vi "Hybrid Get Control Status.vi"(8 "error in (no error)":errorcluster, 11 "VI in":refnum<vi>) -> (0 "error out":errorcluster, 1 "Pause":bool, 2 "Ramp":bool, 3 "VI out":refnum<vi>, 5 "Slew Rate [A/s]":dbl format="%.1f", 7 "Setpoint":dbl format="%.2f")   [LabVIEW 2019]
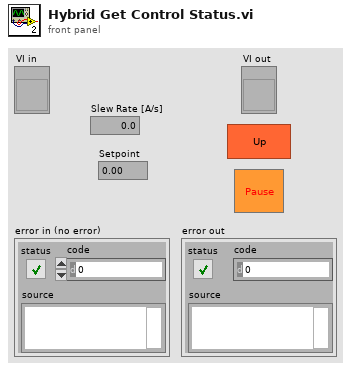
[diagram p1: front panel]
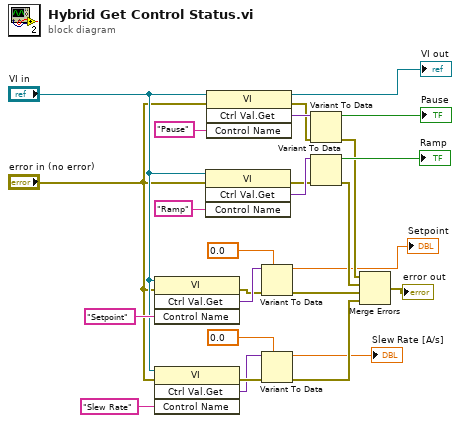
[diagram p0: block diagram]
diagram:
  n1 = invoke class="VI" method="Ctrl Val.Get"(reference="VI in", error in="error in (no error)", "Control Name"="Setpoint") -> (error out=w15:errorcluster, "Get Control Value Variant"=w16:variant)  [unwired: 1 in, 2 out]
  n2 = invoke class="VI" method="Ctrl Val.Get"(reference="VI in", error in="error in (no error)", "Control Name"="Slew Rate") -> (error out=w14:errorcluster, "Get Control Value Variant"=w13:variant)  [unwired: 1 in, 2 out]
  n3 = invoke class="VI" method="Ctrl Val.Get"(reference="VI in", error in="error in (no error)", "Control Name"="Ramp") -> (error out=w6:errorcluster, "Get Control Value Variant"=w22:variant)  [unwired: 1 in, 2 out]
  n4 = invoke class="VI" method="Ctrl Val.Get"(reference="VI in", error in="error in (no error)", "Control Name"="Pause") -> (reference out=→"VI out":refnum<vi>, error out=w5:errorcluster, "Get Control Value Variant"=w21:variant)  [unwired: 1 in, 1 out]
  n5 = Variant To Data(error in=w15, type=0.0 ("Current [KA]"), Variant=w16) -> (data=→"Setpoint":dbl, error out=w4:errorcluster)
  n6 = Variant To Data(error in=w14, type=0.0 ("Current [KA]"), Variant=w13) -> (data=→"Slew Rate [A/s]":dbl, error out=w3:errorcluster)
  n7 = Variant To Data(error in=w5, Variant=w21) -> (data=→"Pause":bool, error out=w8:errorcluster)  [unwired: 1 in]
  n8 = Variant To Data(error in=w6, Variant=w22) -> (data=→"Ramp":bool, error out=w7:errorcluster)  [unwired: 1 in]
  n9 = Merge Errors(w8, w7, w4, w3) -> (→"error out":errorcluster)
